vi "LSX Set Snapshot Par.vi"(8 "error in (no error)":errorcluster, 9 "bAutoMode":i32, 10 "bHigh":i32, 11 "lLSID":i32) -> (0 "error out":errorcluster, 3 "function return":i32)   [LabVIEW 2018, in "Tango.lvlib"]
doc: "TANGOAPI int TANGOCALL LSX_SetSnapshotPar (int lLSID, BOOL bHigh, BOOL bAutoMode);"
uses:
  <userlib>/Tango/Tango.lvlib
  <userlib>/Tango/Tango_DLL.dll
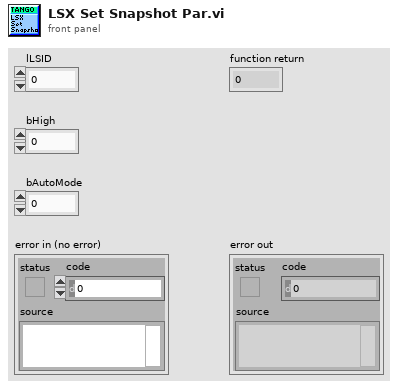
[diagram p1: front panel]
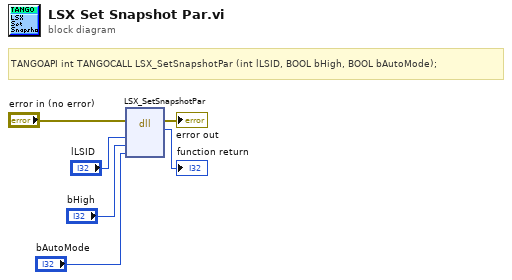
[diagram p0: block diagram]
diagram:
  # "TANGOAPI int TANGOCALL LSX_SetSnapshotPar (int lLSID, BOOL bHigh, BOOL bAutoMode);"
  n1 = dll-call lib="C:/Program Files (x86)/National Instruments/LabVIEW 2018/user.lib/Tango/Tango_DLL.*" fn="LSX_SetSnapshotPar"(error in="error in (no error)", "lLSID"="lLSID", "bHigh"="bHigh", "bAutoMode"="bAutoMode") -> (error out=→"error out":errorcluster, →"function return":i32)  [unwired: 5 in, 1 out]
